vi "set max time.vi"(1 "stopping criteria":T2={"function tolerance"=1e-06, "parameter tolerance"=1e-06, "max iterations"=100, "max function calls"=1000, "gradient tolerance"=1e-06, "max time (sec)"=1000.0}) -> (0 "stopping criteria":T1={"function tolerance"=1e-06, "parameter tolerance"=1e-06, "max iterations"=0, "max function calls"=0, "gradient tolerance"=0.0, "max time (sec)"=1000.0, "initial tick count"=0})   [LabVIEW 2017, in "NI_Gmath.lvlib"]
uses:
  NI_Gmath.lvlib
  stopping criteria.ctl
  stopping criteria with time.ctl
panel:
  in  "stopping criteria 2":T1={"function tolerance"=1e-06, "parameter tolerance"=1e-06, "max iterations"=0, "max function calls"=0, "gradient tolerance"=0.0, "max time (sec)"=1000.0, "initial tick count"=0}
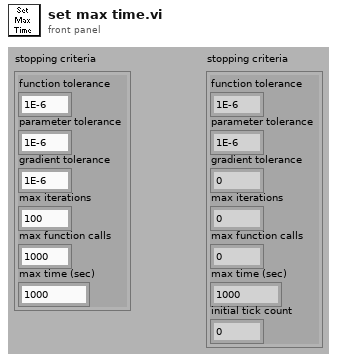
[diagram p1: front panel]
types:
  T1 = typedef "NI_Gmath.lvlib/stopping criteria with time.ctl" = cluster{"function tolerance":dbl, "parameter tolerance":dbl, "max iterations":i32, "max function calls":i32, "gradient tolerance":dbl, "max time (sec)":dbl, "initial tick count":u32}
  T2 = typedef "NI_Gmath.lvlib/stopping criteria.ctl" = cluster{"function tolerance":dbl, "parameter tolerance":dbl, "max iterations":i32, "max function calls":i32, "gradient tolerance":dbl, "max time (sec)":dbl}
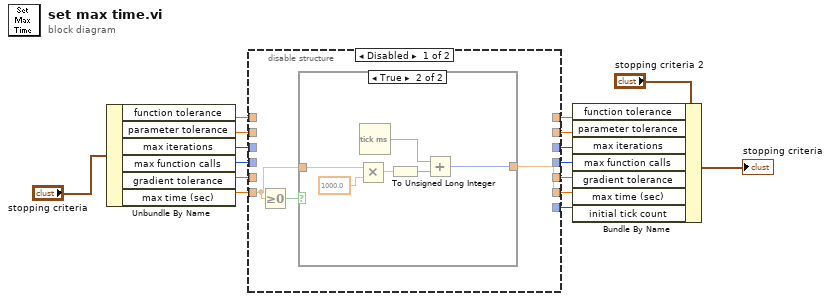
[diagram p0: block diagram]
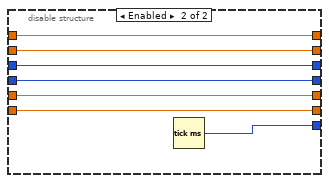
[diagram p3: hidden frame]
diagram:
  n1 = Unbundle By Name("stopping criteria") -> ("function tolerance"=w2:dbl, "parameter tolerance"=w4:dbl, "max iterations"=w6:i32, "max function calls"=w8:i32, "gradient tolerance"=w10:dbl, "max time (sec)"=w14:dbl)
  n2 = disable-structure shown="Disabled" {
    disable-tunnel: [w19 w32] -> w16
    disable-tunnel: w14 -> [w18 w32]
    disable-tunnel: [_ w33] -> w12
    disable-tunnel: [_ w31] -> w11
    disable-tunnel: w10 -> [_ w31]
    disable-tunnel: [_ w30] -> w9
    disable-tunnel: w8 -> [_ w30]
    disable-tunnel: [_ w29] -> w7
    disable-tunnel: w6 -> [_ w29]
    disable-tunnel: [_ w28] -> w5
    disable-tunnel: w4 -> [_ w28]
    disable-tunnel: [_ w27] -> w3
    disable-tunnel: w2 -> [_ w27]
    frame Disabled {
      n3 = Greater Or Equal To 0?(x=w18) -> (x >= 0?=w17:bool)
      n4 = case shown="True" w17 {
        tunnel: w18 -> [w20 w23]
        tunnel: [w20 w22] -> w19
        frame False {
        }
        frame True {
          n5 = Multiply(x=w23, y=1000.0) -> (x*y=w25:dbl)
          n6 = Tick Count (ms)() -> (millisecond timer value=w24:u32)
          n7 = To Unsigned Long Integer(number=w25) -> (unsigned 32bit integer=w21:u32)
          n8 = Add(x=w24, y=w21) -> (x+y=w22:u32)
        }
      }
    }
    frame Enabled {
      n9 = Tick Count (ms)() -> (millisecond timer value=w33:u32)
    }
  }
  n10 = Bundle By Name(cluster="stopping criteria 2", "function tolerance"=w3, "parameter tolerance"=w5, "max iterations"=w7, "max function calls"=w9, "gradient tolerance"=w11, "max time (sec)"=w16, "initial tick count"=w12) -> (→"stopping criteria":T1)
